vi "OAT Decimate Filter Specification.vi"(7 "alias free":bool, 10 "bandwidth":cluster{"passband":dbl, "stopband":dbl} {"stopband" format="%.2f"; "passband" format="%.2f"}, 11 "interpolation/decimation factor":i32=2) -> (2 "bandwidth":cluster{"passband":dbl, "stopband":dbl} {"stopband" format="%.2f"; "passband" format="%.2f"}, 3 "current factor":i32=2)   [LabVIEW 2017, in "SoundVib_Resampling.lvlib"]
uses:
  <vilib>/addons/Sound and Vibration/Order Analysis/Resample Order Tracking/SoundVib_Resampling.lvlib
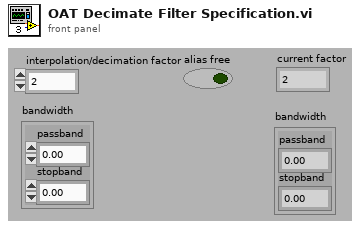
[diagram p1: front panel]
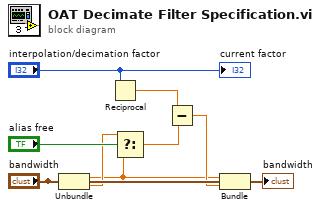
[diagram p0: block diagram]
diagram:
  n1 = Unbundle("bandwidth") -> ("passband"=w2:dbl, "stopband"=w4:dbl)
  n2 = Reciprocal(x="interpolation/decimation factor") -> (1/x=w8:dbl)
  n3 = Select(t=w4, s="alias free", f=w2) -> (s? t:f=w7:dbl)
  n4 = Subtract(x=w8, y=w7) -> (x-y=w3:dbl)
  n5 = Bundle(cluster="bandwidth", "passband"=w2, "stopband"=w3) -> (→"bandwidth":cluster{"passband":dbl, "stopband":dbl})
  "current factor" <- "interpolation/decimation factor"
